vi "Cleanup.vi"(8 "error in (no error)":errorcluster, 11 "WebServer in":refnum<class "WebServer.lvclass">) -> (0 "error out":errorcluster)   [LabVIEW 2022 SP3, in "VMR-Deck.lvlib" / "WebServer.lvclass"]
uses:
  WebServer.lvclass
  WebServer.lvclass/WebServer.ctl
  <vilib>/IlluminatedG/IG HTTP Server/HTTP Server/Server/Server.lvclass
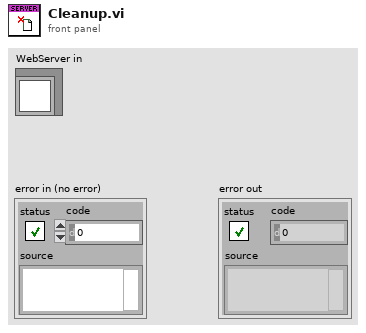
[diagram p1: front panel]
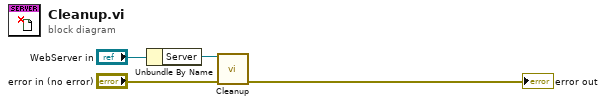
[diagram p0: block diagram]
diagram:
  n1 = Unbundle By Name("WebServer in") -> ("Server"=w2:refnum<class "Server.lvclass">)
  n2 = call <vilib>:"Cleanup.vi"("error in (no error)"="error in (no error)", "Server in"=w2) -> ("error out"=→"error out":errorcluster)  [unwired: 9 in]
